vi "Lab Panel V4.83.vi"() -> ()   [LabVIEW 2013] (continued)
            n215 = property on="Network Directory" class="Path"("Blinking"=w253) -> ()  [unwired: 2 in, 2 out]
            n216 = property on="Message" class="Str"("Blinking"=w253) -> ()  [unwired: 2 in, 2 out]
          }
        }
        frame #10 {
          w261 = FALSE
          n217 = property on="Message" class="Str"("Blinking"=w261) -> ()  [unwired: 2 in, 2 out]
          n218 = property on="Network Directory" class="Path"("Blinking"=w261) -> ()  [unwired: 2 in, 2 out]
          n219 = property on="Tab Control 2" class="TabCtl (strict)"("Value"=0) -> ()  [unwired: 2 in, 2 out]
        }
      }
    }
    frame #2 {
      n220 = node-c288("loop  delay(mS)") -> (w265:T15)  [unwired: 3 in]
      n221 = timed-loop {
        timing: w265 -> [_]
        timing-out: [_] -> w264
        i -> [w287]
        stop <- "stop" stop-if-true
        n222 = node-c288() -> ()  [unwired: 1 in, 1 out]
        n223 = global write "Global display 1.vi" "stop disp"("stop") -> ()
        n224 = local read "SELECT LAB05-2"() -> (w267:T3)
        n225 = local read "SELECT LAB05-1"() -> (w268:T3)
        n226 = local read "SELECT LAB04-2"() -> (w269:T3)
        n227 = local read "SELECT LAB03-1"() -> (w272:T3)
        n228 = local read "SELECT LAB02-2"() -> (w273:T3)
        n229 = local read "SELECT LAB01-1"() -> (w276:T3)
        n230 = local read "SELECT LAB03-2"() -> (w271:T3)
        n231 = local read "SELECT LAB01-2"() -> (w275:T3)
        n232 = local read "SELECT LAB04-1"() -> (w270:T3)
        n233 = local read "SELECT LAB02-1"() -> (w274:T3)
        n234 = local read "run lab03-2"() -> (w281:bool)
        n235 = local read "run lab04-1"() -> (w280:bool)
        n236 = local read "run lab05-1"() -> (w278:bool)
        n237 = local read "run lab04-2"() -> (w279:bool)
        n238 = local read "run lab05-2"() -> (w277:bool)
        n239 = local read "run lab03-1"() -> (w282:bool)
        n240 = local read "run lab02-2"() -> (w283:bool)
        n241 = local read "run lab02-1"() -> (w284:bool)
        n242 = local read "run lab01-1"() -> (w286:bool)
        n243 = local read "run lab01-2"() -> (w285:bool)
        n244 = stacked-sequence {
          seq-local: [_ w349 _ _ _ _ _ _ _ _ _ _ _ _ _ _ _ _ _ _ _] -> [_ _ _ _ _ w1958 _ _ _ _ _ _ _ _ _ _ _ _ _ _ _]
          seq-local: [_ w348 _ _ _ _ _ _ _ _ _ _ _ _ _ _ _ _ _ _ _] -> [_ _ _ _ _ w1957 _ _ _ _ _ _ _ _ _ _ _ _ _ _ _]
          seq-local: [_ w335 _ _ _ _ _ _ _ _ _ _ _ _ _ _ _ _ _ _ _] -> [_ _ _ _ _ w1956 _ _ _ _ _ _ _ _ _ _ _ _ _ _ _]
          seq-local: [_ w334 _ _ _ _ _ _ _ _ _ _ _ _ _ _ _ _ _ _ _] -> [_ _ _ _ _ w1955 _ _ _ _ _ _ _ _ _ _ _ _ _ _ _]
          seq-local: [_ w333 _ _ _ _ _ _ _ _ _ _ _ _ _ _ _ _ _ _ _] -> [_ _ _ _ _ w1954 _ _ _ _ _ _ _ _ _ _ _ _ _ _ _]
          seq-local: [_ w332 _ _ _ _ _ _ _ _ _ _ _ _ _ _ _ _ _ _ _] -> [_ _ _ _ _ w1953 _ _ _ _ _ _ _ _ _ _ _ _ _ _ _]
          seq-local: [_ w331 _ _ _ _ _ _ _ _ _ _ _ _ _ _ _ _ _ _ _] -> [_ _ _ _ _ w1952 _ _ _ _ _ _ _ _ _ _ _ _ _ _ _]
          seq-local: [_ w330 _ _ _ _ _ _ _ _ _ _ _ _ _ _ _ _ _ _ _] -> [_ _ _ _ _ w1951 _ _ _ _ _ _ _ _ _ _ _ _ _ _ _]
          seq-local: [_ w329 _ _ _ _ _ _ _ _ _ _ _ _ _ _ _ _ _ _ _] -> [_ _ _ _ _ w1950 _ _ _ _ _ _ _ _ _ _ _ _ _ _ _]
          seq-local: [_ w328 _ _ _ _ _ _ _ _ _ _ _ _ _ _ _ _ _ _ _] -> [_ _ _ _ _ w1949 _ _ _ _ _ _ _ _ _ _ _ _ _ _ _]
          tunnel: w286 -> [_ _ w365 w604 w1548 w1978 w2288 w2533 _ _ _ _ w2936 _ w3864 _ _ w4147 w4450 w4623 _]
          tunnel: w285 -> [_ _ w364 w602 w1547 w1977 w2289 w2532 _ _ _ _ w2935 _ w3862 _ _ w4146 w4449 w4621 _]
          tunnel: w284 -> [_ _ w363 w600 w1546 w1976 w2287 w2531 _ _ _ _ w2934 _ w3860 _ _ w4145 w4448 _ _]
          tunnel: w283 -> [_ _ w362 w598 w1545 w1975 w2286 w2530 _ _ _ _ w2933 _ w3858 _ _ w4144 w4447 _ _]
          tunnel: w282 -> [_ _ w361 w596 w1544 w1974 w2285 w2529 _ _ _ _ w2932 _ w3856 _ _ w4143 w4446 _ _]
          tunnel: w281 -> [_ _ w360 w594 w1543 w1973 w2284 w2528 _ _ _ _ w2931 _ w3854 _ _ w4142 w4445 _ _]
          tunnel: w280 -> [_ _ w359 w592 w1542 w1972 w2283 w2527 _ _ _ _ w2930 _ w3852 _ _ w4141 w4444 _ _]
          tunnel: w279 -> [_ _ w358 w590 w1541 w1971 w2282 w2526 _ _ _ _ w2929 _ w3850 _ _ w4140 w4443 _ _]
          tunnel: w278 -> [_ _ w357 w588 w1540 w1970 w2281 w2525 _ _ _ _ w2928 _ w3848 _ _ w4139 w4442 _ _]
          tunnel: w277 -> [_ _ w356 w586 w1539 w1969 w2280 w2524 _ _ _ _ w2927 _ w3846 _ _ w4138 w4441 _ _]
          tunnel: w276 -> [_ _ _ w603 w1538 w1968 _ _ _ _ _ _ _ _ w3866 _ _ _ _ _ _]
          tunnel: w275 -> [_ _ _ w601 w1537 w1967 _ _ _ _ _ _ _ _ w3861 _ _ _ _ _ _]
          tunnel: w274 -> [_ _ _ w599 w1536 w1966 _ _ _ _ _ _ _ _ w3859 _ _ _ _ _ _]
          tunnel: w273 -> [_ _ _ w597 w1535 w1965 _ _ _ _ _ _ _ _ w3857 _ _ _ _ _ _]
          tunnel: w272 -> [_ _ _ w595 w1534 w1964 _ _ _ _ _ _ _ _ w3855 _ _ _ _ _ _]
          tunnel: w271 -> [_ _ _ w593 w1533 w1963 _ _ _ _ _ _ _ _ w3853 _ _ _ _ _ _]
          tunnel: w270 -> [_ _ _ w591 w1532 w1962 _ _ _ _ _ _ _ _ w3851 _ _ _ _ _ _]
          tunnel: w269 -> [_ _ _ w589 w1531 w1961 _ _ _ _ _ _ _ _ w3849 _ _ _ _ _ _]
          tunnel: w268 -> [_ _ _ w587 w1530 w1960 _ _ _ _ _ _ _ _ w3847 _ _ _ _ _ _]
          tunnel: w267 -> [_ _ _ w585 w1529 w1959 _ _ _ _ _ _ _ _ w3845 _ _ _ _ _ _]
          frame #0 {
            w291 = FALSE
            w296 = 0.5
            # "set up cycle control"
            n245 = local read "jig cycle"() -> (w295:dbl)
            n246 = Divide(x="JIG ON TIME (S)", y=w296) -> (x/y=→"on loops":dbl)
            n247 = Divide(x="JIG OFF TIME (S)", y=w296) -> (x/y=→"off loops":dbl)
            n248 = Increment(x=w295) -> (x+1=w294:dbl)
            n249 = local write "TEMP"(w291) -> ()
            n250 = local write "AI"(w291) -> ()
            n251 = local write "jig cycle"(w294) -> ()
            n252 = event shown="[1] \"ADMIN\": Value Change" {
              selector: _ -> [_ _]
              dyn-events: _ -> [_ _]
              timeout: 10 -> [_ _]
              event Timeout {
                n253 = event-data() -> ()  [unwired: 1 in, 3 out]
              }
              event "ADMIN": Value Change {
                n254 = event-data() -> ()  [unwired: 1 in, 6 out]
                n255 = stacked-sequence {
                  seq-local: [_ w300 _] -> [_ _ w301]
                  frame #0 {
                    n256 = global write "Global 1.vi" "password"("9999") -> ()
                  }
                  frame #1 {
                    n257 = call "sub vi - password 1.vi"() -> ("RESULT"=w300:bool)  [unwired: 11 in]
                  }
                  frame #2 {
                    w303 = FALSE
                    n258 = property on="Tab Control 2" class="TabCtl (strict)"() -> ("Pages"=w307:refnum<vi>[])  [unwired: 2 in, 2 out]
                    n259 = Select(t=TRUE, s=w301, f=w303) -> (s? t:f=w302:bool)
                    n260 = Index Array(array=w307, index=9) -> (element=w305:refnum<vi>)
                    n261 = property class="Page"(reference=w305, "PageVis"=w302) -> ()  [unwired: 1 in, 2 out]
                    n262 = local write "ADMIN"(w303) -> ()
                  }
                }
              }
            }
          }
          frame #1 {
            w345 = 60.0
            # "convert temperature rise minutes to cycles"
            n263 = local read "SET LAB05-2"() -> (w309:T5)
            n264 = local read "SET LAB05-1"() -> (w311:T5)
            n265 = local read "SET LAB04-2"() -> (w313:T5)
            n266 = local read "SET LAB01-1"() -> (w327:T5)
            n267 = local read "SET LAB01-2"() -> (w325:T5)
            n268 = local read "SET LAB02-2"() -> (w321:T5)
            n269 = local read "SET LAB04-1"() -> (w315:T5)
            n270 = local read "SET LAB03-1"() -> (w319:T5)
            n271 = local read "SET LAB03-2"() -> (w317:T5)
            n272 = local read "SET LAB02-1"() -> (w323:T5)
            n273 = local read "JIG OFF TIME (S)"() -> (w350:dbl)
            n274 = local read "JIG ON TIME (S)"() -> (w351:dbl)
            n275 = Unbundle(w309) -> ("T-RISE mins"=w308:dbl)  [unwired: 4 out]
            n276 = Unbundle(w311) -> ("T-RISE mins"=w310:dbl)  [unwired: 4 out]
            n277 = Unbundle(w327) -> ("T-RISE mins"=w326:dbl)  [unwired: 4 out]
            n278 = Unbundle(w313) -> ("T-RISE mins"=w312:dbl)  [unwired: 4 out]
            n279 = Unbundle(w325) -> ("T-RISE mins"=w324:dbl)  [unwired: 4 out]
            n280 = Unbundle(w323) -> ("T-RISE mins"=w322:dbl)  [unwired: 4 out]
            n281 = Unbundle(w315) -> ("T-RISE mins"=w314:dbl)  [unwired: 4 out]
            n282 = Unbundle(w321) -> ("T-RISE mins"=w320:dbl)  [unwired: 4 out]
            n283 = Unbundle(w317) -> ("T-RISE mins"=w316:dbl)  [unwired: 4 out]
            n284 = Unbundle(w319) -> ("T-RISE mins"=w318:dbl)  [unwired: 4 out]
            n285 = Add(x=w351, y=w350) -> (x+y=w344:dbl)
            n286 = Multiply(x=w345, y=w316) -> (x*y=w340:dbl)
            n287 = Multiply(x=w345, y=w314) -> (x*y=w339:dbl)
            n288 = Multiply(x=w345, y=w312) -> (x*y=w338:dbl)
            n289 = Multiply(x=w345, y=w310) -> (x*y=w337:dbl)
            n290 = Multiply(x=w345, y=w308) -> (x*y=w336:dbl)
            n291 = Multiply(x=w345, y=w324) -> (x*y=w346:dbl)
            n292 = Multiply(x=w345, y=w318) -> (x*y=w341:dbl)
            n293 = Multiply(x=w345, y=w326) -> (x*y=w347:dbl)
            n294 = Multiply(x=w345, y=w322) -> (x*y=w343:dbl)
            n295 = Multiply(x=w345, y=w320) -> (x*y=w342:dbl)
            n296 = Divide(x=w337, y=w344) -> (x/y=w329:dbl)
            n297 = Divide(x=w338, y=w344) -> (x/y=w330:dbl)
            n298 = Divide(x=w339, y=w344) -> (x/y=w331:dbl)
            n299 = Divide(x=w336, y=w344) -> (x/y=w328:dbl)
            n300 = Divide(x=w341, y=w344) -> (x/y=w333:dbl)
            n301 = Divide(x=w347, y=w344) -> (x/y=w349:dbl)
            n302 = Divide(x=w346, y=w344) -> (x/y=w348:dbl)
            n303 = Divide(x=w343, y=w344) -> (x/y=w335:dbl)
            n304 = Divide(x=w342, y=w344) -> (x/y=w334:dbl)
            n305 = Divide(x=w340, y=w344) -> (x/y=w332:dbl)
          }
          frame #2 {
            # "control cycle loops"
            n306 = local read "JIG OFF TIME (S)"() -> (w354:dbl)
            n307 = local read "JIG ON TIME (S)"() -> (w353:dbl)
            n308 = local read "jig cycle"() -> (w367:dbl)
            n309 = local read "on loops"() -> (w369:dbl)
            n310 = local read "off loops"() -> (w368:dbl)
            n311 = Add(x=w354, y=w353) -> (x+y=w352:dbl)
            n312 = Add(x=w369, y=w368) -> (x+y=w355:dbl)
            n313 = Greater Or Equal?(x=w367, y=w355) -> (x >= y?=w366:bool)
            n314 = case shown="True" w366 {
              tunnel: w365 -> [_ w404]
              tunnel: w364 -> [_ w403]
              tunnel: w363 -> [_ w402]
              tunnel: w362 -> [_ w401]
              tunnel: w361 -> [_ w400]
              tunnel: w360 -> [_ w399]
              tunnel: w359 -> [_ w398]
              tunnel: w358 -> [_ w397]
              tunnel: w357 -> [_ w396]
              tunnel: w356 -> [_ w395]
              tunnel: w352 -> [_ w394]
              frame False {
              }
              frame True {
                # "increment cycle value and convert cycles to minutes for temp rise"
                n315 = local read "Temp Loops"() -> (w371:dbl)
                n316 = local read "JIG RELAY CYCLES"() -> (w393:T7)
                n317 = Increment(x=w371) -> (x+1=w370:dbl)
                n318 = local write "Temp Loops"(w370) -> ()
                n319 = Unbundle By Name(w393) -> ("LAB01-1"=w391:dbl, "LAB01-2"=w389:dbl, "LAB02-1"=w387:dbl, "LAB02-2"=w385:dbl, "LAB03-1"=w383:dbl, "LAB03-2"=w381:dbl, "LAB04-1"=w379:dbl, "LAB04-2"=w377:dbl, "LAB05-1"=w375:dbl, "LAB05-2"=w373:dbl)
                n320 = stacked-sequence {
                  tunnel: w404 -> [w416 _ _ _ _ _ _ _ _ _]
                  tunnel: w403 -> [_ w433 _ _ _ _ _ _ _ _]
                  tunnel: w402 -> [_ _ w450 _ _ _ _ _ _ _]
                  tunnel: w401 -> [_ _ _ w467 _ _ _ _ _ _]
                  tunnel: w400 -> [_ _ _ _ w484 _ _ _ _ _]
                  tunnel: w399 -> [_ _ _ _ _ w501 _ _ _ _]
                  tunnel: w398 -> [_ _ _ _ _ _ w518 _ _ _]
                  tunnel: w397 -> [_ _ _ _ _ _ _ w535 _ _]
                  tunnel: w396 -> [_ _ _ _ _ _ _ _ w552 _]
                  tunnel: w395 -> [_ _ _ _ _ _ _ _ _ w569]
                  tunnel: w394 -> [w413 w430 w447 w464 w481 w498 w515 w532 w549 w566]
                  tunnel: w391 -> [w407 _ _ _ _ _ _ _ _ _]
                  tunnel: [w406 _ _ _ _ _ _ _ _ _] -> w390
                  tunnel: w389 -> [_ w424 _ _ _ _ _ _ _ _]
                  tunnel: [_ w423 _ _ _ _ _ _ _ _] -> w388
                  tunnel: w387 -> [_ _ w441 _ _ _ _ _ _ _]
                  tunnel: [_ _ w440 _ _ _ _ _ _ _] -> w386
                  tunnel: w385 -> [_ _ _ w458 _ _ _ _ _ _]
                  tunnel: [_ _ _ w457 _ _ _ _ _ _] -> w384
                  tunnel: w383 -> [_ _ _ _ w475 _ _ _ _ _]
                  tunnel: [_ _ _ _ w474 _ _ _ _ _] -> w382
                  tunnel: w381 -> [_ _ _ _ _ w492 _ _ _ _]
                  tunnel: [_ _ _ _ _ w491 _ _ _ _] -> w380
                  tunnel: w379 -> [_ _ _ _ _ _ w509 _ _ _]
                  tunnel: [_ _ _ _ _ _ w508 _ _ _] -> w378
                  tunnel: w377 -> [_ _ _ _ _ _ _ w526 _ _]
                  tunnel: [_ _ _ _ _ _ _ w525 _ _] -> w376
                  tunnel: w375 -> [_ _ _ _ _ _ _ _ w543 _]
                  tunnel: [_ _ _ _ _ _ _ _ w542 _] -> w374
                  tunnel: w373 -> [_ _ _ _ _ _ _ _ _ w560]
                  tunnel: [_ _ _ _ _ _ _ _ _ w559] -> w372
                  frame #0 {
                    n321 = local read "DISP LAB01-1"() -> (w411:T4)
                    n322 = Unbundle(w411) -> ("CYCLE"=w412:dbl)  [unwired: 2 out]
                    n323 = case shown="True" w416 {
                      tunnel: w412 -> [w418 w422]
                      tunnel: [w418 w421] -> w410
                      tunnel: w407 -> [w417 w420]
                      tunnel: [w417 w419] -> w406
                      frame False {
                      }
                      frame True {
                        n324 = Increment(x=w420) -> (x+1=w419:dbl)
                        n325 = Increment(x=w422) -> (x+1=w421:dbl)
                      }
                    }
                    n326 = Multiply(x=w410, y=w413) -> (x*y=w414:dbl)
                    n327 = Divide(x=w414, y=60.0) -> (x/y=w409:dbl)
                    n328 = Bundle(cluster=w411, "CYCLE"=w410, "MINS"=w409) -> (w408:T4)  [unwired: 1 in]
                    n329 = local write "DISP LAB01-1"(w408) -> ()
                  }
                  frame #1 {
                    n330 = local read "DISP LAB01-2"() -> (w428:T4)
                    n331 = Unbundle(w428) -> ("CYCLE"=w429:dbl)  [unwired: 2 out]
                    n332 = case shown="True" w433 {
                      tunnel: w429 -> [w435 w439]
                      tunnel: [w435 w438] -> w426
                      tunnel: w424 -> [w434 w437]
                      tunnel: [w434 w436] -> w423
                      frame False {
                      }
                      frame True {
                        n333 = Increment(x=w437) -> (x+1=w436:dbl)
                        n334 = Increment(x=w439) -> (x+1=w438:dbl)
                      }
                    }
                    n335 = Multiply(x=w426, y=w430) -> (x*y=w431:dbl)
                    n336 = Divide(x=w431, y=60.0) -> (x/y=w425:dbl)
                    n337 = Bundle(cluster=w428, "CYCLE"=w426, "MINS"=w425) -> (w427:T4)  [unwired: 1 in]
                    n338 = local write "DISP LAB01-2"(w427) -> ()
                  }
                  frame #2 {
                    n339 = local read "DISP LAB02-1"() -> (w445:T4)
                    n340 = Unbundle(w445) -> ("CYCLE"=w446:dbl)  [unwired: 2 out]
                    n341 = case shown="True" w450 {
                      tunnel: [w452 w456] -> w443
                      tunnel: w446 -> [w452 w455]
                      tunnel: w441 -> [w451 w454]
                      tunnel: [w451 w453] -> w440
                      frame False {
                      }
                      frame True {
                        n342 = Increment(x=w454) -> (x+1=w453:dbl)
                        n343 = Increment(x=w455) -> (x+1=w456:dbl)
                      }
                    }
                    n344 = Multiply(x=w443, y=w447) -> (x*y=w448:dbl)
                    n345 = Divide(x=w448, y=60.0) -> (x/y=w442:dbl)
                    n346 = Bundle(cluster=w445, "CYCLE"=w443, "MINS"=w442) -> (w444:T4)  [unwired: 1 in]
                    n347 = local write "DISP LAB02-1"(w444) -> ()
                  }
                  frame #3 {
                    n348 = local read "DISP LAB02-2"() -> (w462:T4)
                    n349 = Unbundle(w462) -> ("CYCLE"=w463:dbl)  [unwired: 2 out]
                    n350 = case shown="True" w467 {
                      tunnel: [w469 w473] -> w461
                      tunnel: w463 -> [w469 w472]
                      tunnel: w458 -> [w468 w471]
                      tunnel: [w468 w470] -> w457
                      frame False {
                      }
                      frame True {
                        n351 = Increment(x=w471) -> (x+1=w470:dbl)
                        n352 = Increment(x=w472) -> (x+1=w473:dbl)
                      }
                    }
                    n353 = Multiply(x=w461, y=w464) -> (x*y=w465:dbl)
                    n354 = Divide(x=w465, y=60.0) -> (x/y=w460:dbl)
                    n355 = Bundle(cluster=w462, "CYCLE"=w461, "MINS"=w460) -> (w459:T4)  [unwired: 1 in]
                    n356 = local write "DISP LAB02-2"(w459) -> ()
                  }
                  frame #4 {
                    n357 = local read "DISP LAB03-1"() -> (w479:T4)
                    n358 = Unbundle(w479) -> ("CYCLE"=w480:dbl)  [unwired: 2 out]
                    n359 = case shown="True" w484 {
                      tunnel: [w486 w490] -> w476
                      tunnel: w480 -> [w486 w489]
                      tunnel: w475 -> [w485 w488]
                      tunnel: [w485 w487] -> w474
                      frame False {
                      }
                      frame True {
                        n360 = Increment(x=w488) -> (x+1=w487:dbl)
                        n361 = Increment(x=w489) -> (x+1=w490:dbl)
                      }
                    }
                    n362 = Multiply(x=w476, y=w481) -> (x*y=w482:dbl)
                    n363 = Divide(x=w482, y=60.0) -> (x/y=w477:dbl)
                    n364 = Bundle(cluster=w479, "CYCLE"=w476, "MINS"=w477) -> (w478:T4)  [unwired: 1 in]
                    n365 = local write "DISP LAB03-1"(w478) -> ()
                  }
                  frame #5 {
                    n366 = local read "DISP LAB03-2"() -> (w496:T4)
                    n367 = Unbundle(w496) -> ("CYCLE"=w497:dbl)  [unwired: 2 out]
                    n368 = case shown="True" w501 {
                      tunnel: [w503 w507] -> w495
                      tunnel: w497 -> [w503 w506]
                      tunnel: w492 -> [w502 w505]
                      tunnel: [w502 w504] -> w491
                      frame False {
                      }
                      frame True {
                        n369 = Increment(x=w505) -> (x+1=w504:dbl)
                        n370 = Increment(x=w506) -> (x+1=w507:dbl)
                      }
                    }
                    n371 = Multiply(x=w495, y=w498) -> (x*y=w499:dbl)
                    n372 = Divide(x=w499, y=60.0) -> (x/y=w494:dbl)
                    n373 = Bundle(cluster=w496, "CYCLE"=w495, "MINS"=w494) -> (w493:T4)  [unwired: 1 in]
                    n374 = local write "DISP LAB03-2"(w493) -> ()
                  }
                  frame #6 {
                    n375 = local read "DISP LAB04-1"() -> (w513:T4)
                    n376 = Unbundle(w513) -> ("CYCLE"=w514:dbl)  [unwired: 2 out]
                    n377 = case shown="True" w518 {
                      tunnel: [w520 w524] -> w511
                      tunnel: w514 -> [w520 w523]
                      tunnel: w509 -> [w519 w522]
                      tunnel: [w519 w521] -> w508
                      frame False {
                      }
                      frame True {
                        n378 = Increment(x=w522) -> (x+1=w521:dbl)
                        n379 = Increment(x=w523) -> (x+1=w524:dbl)
                      }
                    }
                    n380 = Multiply(x=w511, y=w515) -> (x*y=w516:dbl)
                    n381 = Divide(x=w516, y=60.0) -> (x/y=w510:dbl)
                    n382 = Bundle(cluster=w513, "CYCLE"=w511, "MINS"=w510) -> (w512:T4)  [unwired: 1 in]
                    n383 = local write "DISP LAB04-1"(w512) -> ()
                  }
                  frame #7 {
                    n384 = local read "DISP LAB04-2"() -> (w530:T4)
                    n385 = Unbundle(w530) -> ("CYCLE"=w531:dbl)  [unwired: 2 out]
                    n386 = case shown="True" w535 {
                      tunnel: [w537 w541] -> w528
                      tunnel: w531 -> [w537 w540]
                      tunnel: w526 -> [w536 w539]
                      tunnel: [w536 w538] -> w525
                      frame False {
                      }
                      frame True {
                        n387 = Increment(x=w539) -> (x+1=w538:dbl)
                        n388 = Increment(x=w540) -> (x+1=w541:dbl)
                      }
                    }
                    n389 = Multiply(x=w528, y=w532) -> (x*y=w534:dbl)
                    n390 = Divide(x=w534, y=60.0) -> (x/y=w527:dbl)
                    n391 = Bundle(cluster=w530, "CYCLE"=w528, "MINS"=w527) -> (w529:T4)  [unwired: 1 in]
                    n392 = local write "DISP LAB04-2"(w529) -> ()
                  }
                  frame #8 {
                    n393 = local read "DISP LAB05-1"() -> (w547:T4)
                    n394 = Unbundle(w547) -> ("CYCLE"=w548:dbl)  [unwired: 2 out]
                    n395 = case shown="True" w552 {
                      tunnel: [w554 w558] -> w545
                      tunnel: w548 -> [w554 w557]
                      tunnel: w543 -> [w553 w556]
                      tunnel: [w553 w555] -> w542
                      frame False {
                      }
                      frame True {
                        n396 = Increment(x=w556) -> (x+1=w555:dbl)
                        n397 = Increment(x=w557) -> (x+1=w558:dbl)
                      }
                    }
                    n398 = Multiply(x=w545, y=w549) -> (x*y=w550:dbl)
                    n399 = Divide(x=w550, y=60.0) -> (x/y=w544:dbl)
                    n400 = Bundle(cluster=w547, "CYCLE"=w545, "MINS"=w544) -> (w546:T4)  [unwired: 1 in]
                    n401 = local write "DISP LAB05-1"(w546) -> ()
                  }
                  frame #9 {
                    n402 = local read "DISP LAB05-2"() -> (w565:T4)
                    n403 = Unbundle(w565) -> ("CYCLE"=w564:dbl)  [unwired: 2 out]
                    n404 = case shown="True" w569 {
                      tunnel: [w571 w575] -> w563
                      tunnel: w564 -> [w571 w574]
                      tunnel: w560 -> [w570 w573]
                      tunnel: [w570 w572] -> w559
                      frame False {
                      }
                      frame True {
                        n405 = Increment(x=w573) -> (x+1=w572:dbl)
                        n406 = Increment(x=w574) -> (x+1=w575:dbl)
                      }
                    }
                    n407 = Multiply(x=w563, y=w566) -> (x*y=w567:dbl)
                    n408 = Divide(x=w567, y=60.0) -> (x/y=w562:dbl)
                    n409 = Bundle(cluster=w565, "CYCLE"=w563, "MINS"=w562) -> (w561:T4)  [unwired: 1 in]
                    n410 = local write "DISP LAB05-2"(w561) -> ()
                  }
                }
                n411 = local write "jig cycle"(0) -> ()
                n412 = Bundle By Name(cluster=w393, "LAB01-1"=w390, "LAB01-2"=w388, "LAB02-1"=w386, "LAB02-2"=w384, "LAB03-1"=w382, "LAB03-2"=w380, "LAB04-1"=w378, "LAB04-2"=w376, "LAB05-1"=w374, "LAB05-2"=w372) -> (w392:T7)
                n413 = local write "JIG RELAY CYCLES"(w392) -> ()
              }
            }
          }
          frame #3 {
            # "START & STOP test RUN switch change, start test if true and stop test if false"
            n414 = Get Date/Time In Seconds() -> (seconds since 1Jan1904=w583:timestamp)
            n415 = local read "C drive data root dir"() -> (w576:path)
            n416 = Format Date/Time String(time format string (%c)="%b\\%a%d", seconds (now)=w583) -> (date/time string=w607:string)  [unwired: 1 in]
            n417 = Format Date/Time String(time format string (%c)="%H%M", seconds (now)=w583) -> (date/time string=w605:string)  [unwired: 1 in]
            n418 = Format Date/Time String(time format string (%c)="LabPanel%Y", seconds (now)=w583) -> (date/time string=w582:string)  [unwired: 1 in]
            n419 = Path To String(path=w576) -> (string=w579:string)
            n420 = global write "Global 1.vi" "C drive root path"(w576) -> ()
            n421 = Concatenate Strings(w579, "\\") -> (w577:string)
            n422 = event shown="[5] \"RUN LAB03-1\": Value Change" {
              selector: _ -> [_ _ _ _ _ _ _ _ _ _ _]
              dyn-events: _ -> [_ _ _ _ _ _ _ _ _ _ _]
              timeout: 10 -> [_ _ _ _ _ _ _ _ _ _ _]
              tunnel: w577 -> [_ w615 w707 w799 w891 w983 w1075 w1167 w1259 w1351 w1443]
              tunnel: w607 -> [_ w614 w706 w798 w890 w982 w1074 w1166 w1258 w1350 w1442]
              tunnel: w605 -> [_ w612 w705 w797 w889 w981 w1073 w1165 w1257 w1349 w1441]
              tunnel: w603 -> [_ w613 _ _ _ _ _ _ _ _ _]
              tunnel: w604 -> [_ _ _ _ _ _ _ _ _ _ _]
              tunnel: w602 -> [_ _ _ _ _ _ _ _ _ _ _]
              tunnel: w601 -> [_ _ w704 _ _ _ _ _ _ _ _]
              tunnel: w600 -> [_ _ _ _ _ _ _ _ _ _ _]
              tunnel: w599 -> [_ _ _ w796 _ _ _ _ _ _ _]
              tunnel: w598 -> [_ _ _ _ _ _ _ _ _ _ _]
              tunnel: w597 -> [_ _ _ _ w888 _ _ _ _ _ _]
              tunnel: w596 -> [_ _ _ _ _ _ _ _ _ _ _]
              tunnel: w595 -> [_ _ _ _ _ w980 _ _ _ _ _]
              tunnel: w594 -> [_ _ _ _ _ _ _ _ _ _ _]
              tunnel: w593 -> [_ _ _ _ _ _ w1072 _ _ _ _]
              tunnel: w592 -> [_ _ _ _ _ _ _ _ _ _ _]
              tunnel: w591 -> [_ _ _ _ _ _ _ w1164 _ _ _]
              tunnel: w590 -> [_ _ _ _ _ _ _ _ _ _ _]
              tunnel: w589 -> [_ _ _ _ _ _ _ _ w1256 _ _]
              tunnel: w588 -> [_ _ _ _ _ _ _ _ _ _ _]
              tunnel: w587 -> [_ _ _ _ _ _ _ _ _ w1348 _]
              tunnel: w586 -> [_ _ _ _ _ _ _ _ _ _ _]
              tunnel: w585 -> [_ _ _ _ _ _ _ _ _ _ w1440]
              tunnel: w582 -> [_ w611 w703 w795 w887 w979 w1071 w1163 w1255 w1347 w1439]
              tunnel: [_ w610 w702 w794 w886 w978 w1070 w1162 w1254 w1346 w1438] -> w580
              event Timeout {
                n423 = event-data() -> ()  [unwired: 1 in, 3 out]
              }
              event "RUN LAB01-1": Value Change {
                n424 = event-data() -> ("NewVal"=w609:bool)  [unwired: 1 in, 5 out]
                n425 = local write "run lab01-1"(w609) -> ()
                n426 = case shown="True" w609 {
                  tunnel: w615 -> [_ w648]
                  tunnel: w614 -> [_ w647]
                  tunnel: w613 -> [w617 w646]
                  tunnel: w612 -> [_ w645]
                  tunnel: w611 -> [_ w644]
                  tunnel: [w616 w643] -> w610
                  frame False {
                    # "stop test"
                    n427 = stacked-sequence {
                      tunnel: w617 -> [_ w629 _ _]
                      tunnel: [_ w621 _ _] -> w616
                      frame #0 {
                        n428 = local read "DISP LAB01-1"() -> (w620:T4)
                        n429 = Bundle(cluster=w620, "STATUS"="STOP") -> (w618:T4)  [unwired: 2 in]
                        n430 = local write "DISP LAB01-1"(w618) -> ()
                      }
                      frame #1 {
                        n431 = local read "DISP LAB01-1"() -> (w628:T4)
                        n432 = Unbundle(w628) -> ("CYCLE"=w626:dbl, "MINS"=w627:dbl)  [unwired: 1 out]
                        n433 = case shown="\"CYCLE TEST\"" w629 {
                          tunnel: w627 -> [_ _ w636]
                          tunnel: w626 -> [w634 w635 _]
                          tunnel: [w634 w635 w636] -> w625
                          frame "CHART TEST", Default {
                          }
                          frame "CYCLE TEST" {
                          }
                          frame "T-RISE TEST" {
                          }
                        }
                        n434 = local read "TDMS LAB01-1"() -> (w633:refnum<k34>)
                        n435 = Build Array("STOPPED") -> (w630:string[])
                        n436 = Build Array(w625) -> (w624:dbl[])
                        n437 = TDMS Write(0:w633, 5:"TEST RESULT", 7:w630, 9:w624) -> (4:w622:refnum<k34>, 15:w623:errorcluster)  [unwired: 2 in, 2 out]
                        n438 = TDMS Close(8:w623, 11:w622) -> (0:w621:errorcluster)  [unwired: 1 out]
                      }
                      frame #2 {
                        n439 = stacked-sequence {
                          tunnel: "LAB01-1" -> [w639 w641]
                          frame #0 {
                            n440 = call "sub vi - defrag tdms v1.vi"("panel id"=w639) -> ("error out"=w638:errorcluster)  [unwired: 10 in]
                            n441 = local write "data file error"(w638) -> ()
                          }
                          frame #1 {
                            n442 = call "Save data file to network drive v1.vi"("panel id"=w641) -> ("network file save error"=w640:errorcluster)  [unwired: 9 in, 1 out]
                            n443 = local write "RESULT LAB01-1"(FALSE) -> ()
                            n444 = local write "data file error"(w640) -> ()
                          }
                        }
                      }
                      frame #3 {
                      }
                    }
                  }
                  frame True {
                    # "start new test and create test file"
                    n445 = stacked-sequence {
                      seq-local: [w649 _ _ _ _] -> [_ w670 _ _ _]
                      tunnel: w648 -> [w654 _ _ _ _]
                      tunnel: w647 -> [w650 _ _ _ _]
                      tunnel: w646 -> [w664 _ _ _ _]
                      tunnel: w645 -> [w657 _ _ _ _]
                      tunnel: w644 -> [w652 _ _ _ _]
                      tunnel: [_ w671 _ _ _] -> w643
                      frame #0 {
                        w651 = "\\"
                        n446 = case shown="\"CHART TEST\", Default" w664 {
                          tunnel: ["L01-1-CHART TEST-" "L01-1-CYCLE TEST-" "L01-1-T-RISE TEST-"] -> w660
                          frame "CHART TEST", Default {
                          }
                          frame "CYCLE TEST" {
                          }
                          frame "T-RISE TEST" {
                          }
                        }
                        n447 = local read "SET LAB01-1"() -> (w659:T5)
                        n448 = Unbundle(w659) -> ("DESCRIPTION"=w658:string)  [unwired: 4 out]
                        n449 = Concatenate Strings(w654, "\\", w652, w651, w650, w651) -> (w661:string)
                        n450 = String To Path(string=w661) -> (path=w663:path)
                        n451 = Concatenate Strings(w661, w660, w658, "-", w657, ".tdms") -> (w649:string)
                        n452 = Create Folder(path (use dialog)=w663) -> (error out=w662:errorcluster)  [unwired: 2 in, 2 out]
                        n453 = call <vilib>:"Clear Errors.vi"("error in (no error)"=w662) -> ()  [unwired: 6 in, 1 out]
                        n454 = global write "Global 1.vi" "LAB01-1 FILE"(w649) -> ()
                      }
                      frame #1 {
                        n455 = String To Path(string=w670) -> (path=w668:path)
                        n456 = TDMS Open(5:FALSE, 6:FALSE, 10:T18."create or replace" ("operation (0:open)"), 11:w668) -> (0:w671:errorcluster, 3:→"TDMS LAB01-1":refnum<k34>)  [unwired: 3 in]
                      }
                      frame #2 {
                        n457 = local read "TDMS LAB01-1"() -> (w691:refnum<k34>)
                        n458 = local read "SET LAB01-1"() -> (w680:T5)
                        n459 = Build Array("Testers Name", "Description", "Set Test Cycles", "T-Rise minutes", "T-Rise Deg C") -> (w681:string[])
                        n460 = Unbundle(w680) -> ("NAME"=w679:string, "DESCRIPTION"=w678:string, "CYCLES"=w677:dbl, "T-RISE mins"=w676:dbl, "T-RISE deg C"=w675:dbl)
                        n461 = Number To Decimal String(number=w677) -> (decimal integer string=w690:string)  [unwired: 1 in]
                        n462 = Number To Decimal String(number=w676) -> (decimal integer string=w689:string)  [unwired: 1 in]
                        n463 = Number To Decimal String(number=w675) -> (decimal integer string=w688:string)  [unwired: 1 in]
                        n464 = Build Array(w679, w678, w690, w689, w688) -> (w687:string[])
                        n465 = TDMS Set Properties(5:w687, 7:w681, 11:w691) -> ()  [unwired: 3 in, 4 out]
                      }
                      frame #3 {
                        w692 = 0.0
                        n466 = local read "DISP LAB01-1"() -> (w695:T4)
                        n467 = Bundle(cluster=w695, "CYCLE"=w692, "MINS"=w692, "STATUS"="RUN") -> (w694:T4)
                        n468 = local write "DISP LAB01-1"(w694) -> ()
                      }
                      frame #4 {
                        n469 = local read "SIG LAB01-1"() -> (w698:T2)
                        n470 = local read "TEMP START LAB01-1"() -> (w700:cluster{"TL":dbl, "TN":dbl})
                        n471 = Unbundle(w698) -> ("Tmp Live"=w697:dbl, "Tmp Neut"=w696:dbl)  [unwired: 3 out]
                        n472 = Bundle(cluster=w700, "TL"=w697, "TN"=w696) -> (w699:cluster{"TL":dbl, "TN":dbl})
                        n473 = local write "TEMP START LAB01-1"(w699) -> ()
                      }
                    }
                  }
                }
              }
              event "RUN LAB01-2": Value Change {
                n474 = event-data() -> ("NewVal"=w701:bool)  [unwired: 1 in, 5 out]
                n475 = local write "run lab01-2"(w701) -> ()
                n476 = case shown="True" w701 {
                  tunnel: w707 -> [_ w740]
                  tunnel: w706 -> [_ w739]
                  tunnel: w704 -> [w709 w738]
                  tunnel: w705 -> [_ w737]
                  tunnel: w703 -> [_ w736]
                  tunnel: [w708 w735] -> w702
                  frame False {
                    # "stop test"
                    n477 = stacked-sequence {
                      tunnel: w709 -> [w718 _]
                      tunnel: [w710 _] -> w708
                      frame #0 {
                        n478 = local read "DISP LAB01-2"() -> (w717:T4)
                        n479 = Unbundle(w717) -> ("CYCLE"=w715:dbl, "MINS"=w716:dbl)  [unwired: 1 out]
                        n480 = case shown="\"CHART TEST\", Default" w718 {
                          tunnel: w716 -> [_ _ w725]
                          tunnel: w715 -> [w723 w724 _]
                          tunnel: [w723 w724 w725] -> w714
                          frame "CHART TEST", Default {
                          }
                          frame "CYCLE TEST" {
                          }
                          frame "T-RISE TEST" {
                          }
                        }
                        n481 = local read "TDMS LAB01-2"() -> (w722:refnum<k34>)
                        n482 = Build Array("STOPPED") -> (w719:string[])
                        n483 = Build Array(w714) -> (w713:dbl[])
                        n484 = TDMS Write(0:w722, 5:"TEST RESULT", 7:w719, 9:w713) -> (4:w711:refnum<k34>, 15:w712:errorcluster)  [unwired: 2 in, 2 out]
                        n485 = TDMS Close(8:w712, 11:w711) -> (0:w710:errorcluster)  [unwired: 1 out]
                      }
                      frame #1 {
                        n486 = local read "DISP LAB01-2"() -> (w729:T4)
                        n487 = stacked-sequence {
                          tunnel: "LAB01-2" -> [w731 w733]
                          frame #0 {
                            n488 = call "sub vi - defrag tdms v1.vi"("panel id"=w731) -> ("error out"=w730:errorcluster)  [unwired: 10 in]
                            n489 = local write "data file error"(w730) -> ()
                          }
                          frame #1 {
                            n490 = call "Save data file to network drive v1.vi"("panel id"=w733) -> ("network file save error"=w732:errorcluster)  [unwired: 9 in, 1 out]
                            n491 = local write "RESULT LAB01-2"(FALSE) -> ()
                            n492 = local write "data file error"(w732) -> ()
                          }
                        }
                        n493 = Bundle(cluster=w729, "STATUS"="STOP") -> (w727:T4)  [unwired: 2 in]
                        n494 = local write "DISP LAB01-2"(w727) -> ()
                      }
                    }
                  }
                  frame True {
                    # "start new test and create test file"
                    n495 = stacked-sequence {
                      seq-local: [w741 _ _ _ _] -> [_ w766 _ _ _]
                      tunnel: w740 -> [w746 _ _ _ _]
                      tunnel: w739 -> [w743 _ _ _ _]
                      tunnel: w738 -> [w756 _ _ _ _]
                      tunnel: w737 -> [w749 _ _ _ _]
                      tunnel: w736 -> [w744 _ _ _ _]
                      tunnel: [_ w760 _ _ _] -> w735
                      frame #0 {
                        w742 = "\\"
                        n496 = local read "SET LAB01-2"() -> (w751:T5)
                        n497 = case shown="\"CYCLE TEST\"" w756 {
                          tunnel: ["L01-2-CHART TEST-" "L01-2-CYCLE TEST-" "L01-2-T-RISE TEST-"] -> w752
                          frame "CHART TEST", Default {
                          }
                          frame "CYCLE TEST" {
                          }
                          frame "T-RISE TEST" {
                          }
                        }
                        n498 = Unbundle(w751) -> ("DESCRIPTION"=w750:string)  [unwired: 4 out]
                        n499 = Concatenate Strings(w746, "\\", w744, w742, w743, w742) -> (w753:string)
                        n500 = String To Path(string=w753) -> (path=w755:path)
                        n501 = Concatenate Strings(w753, w752, w750, "-", w749, ".tdms") -> (w741:string)
                        n502 = Create Folder(path (use dialog)=w755) -> (error out=w754:errorcluster)  [unwired: 2 in, 2 out]
                        n503 = global write "Global 1.vi" "LAB01-2 FILE"(w741) -> ()
                        n504 = call <vilib>:"Clear Errors.vi"("error in (no error)"=w754) -> ()  [unwired: 6 in, 1 out]
                      }
                      frame #1 {
                        n505 = String To Path(string=w766) -> (path=w761:path)
                        n506 = TDMS Open(5:FALSE, 6:FALSE, 10:T18."create or replace" ("operation (0:open)"), 11:w761) -> (0:w760:errorcluster, 3:→"TDMS LAB01-2":refnum<k34>)  [unwired: 3 in]
                      }
                      frame #2 {
                        n507 = local read "SET LAB01-2"() -> (w772:T5)
                        n508 = local read "TDMS LAB01-2"() -> (w783:refnum<k34>)
                        n509 = Build Array("Testers Name", "Description", "Set Test Cycles", "T-Rise minutes", "T-Rise Deg C") -> (w773:string[])
                        n510 = Unbundle(w772) -> ("NAME"=w771:string, "DESCRIPTION"=w770:string, "CYCLES"=w769:dbl, "T-RISE mins"=w768:dbl, "T-RISE deg C"=w767:dbl)
                        n511 = Number To Decimal String(number=w769) -> (decimal integer string=w782:string)  [unwired: 1 in]
                        n512 = Number To Decimal String(number=w768) -> (decimal integer string=w781:string)  [unwired: 1 in]
                        n513 = Number To Decimal String(number=w767) -> (decimal integer string=w780:string)  [unwired: 1 in]
                        n514 = Build Array(w771, w770, w782, w781, w780) -> (w779:string[])
                        n515 = TDMS Set Properties(5:w779, 7:w773, 11:w783) -> ()  [unwired: 3 in, 4 out]
                      }
                      frame #3 {
                        w785 = 0.0
                        n516 = local read "DISP LAB01-2"() -> (w787:T4)
                        n517 = Bundle(cluster=w787, "CYCLE"=w785, "MINS"=w785, "STATUS"="RUN") -> (w786:T4)
                        n518 = local write "DISP LAB01-2"(w786) -> ()
                      }
                      frame #4 {
                        n519 = local read "SIG LAB01-2"() -> (w790:T2)
                        n520 = local read "TEMP START LAB01-2"() -> (w792:cluster{"TL":dbl, "TN":dbl})
                        n521 = Unbundle(w790) -> ("Tmp Live"=w789:dbl, "Tmp Neut"=w788:dbl)  [unwired: 3 out]
                        n522 = Bundle(cluster=w792, "TL"=w789, "TN"=w788) -> (w791:cluster{"TL":dbl, "TN":dbl})
                        n523 = local write "TEMP START LAB01-2"(w791) -> ()
                      }
                    }
                  }
                }
              }
              event "RUN LAB02-1": Value Change {
                n524 = event-data() -> ("NewVal"=w793:bool)  [unwired: 1 in, 5 out]
                n525 = local write "run lab02-1"(w793) -> ()
                n526 = case shown="True" w793 {
                  tunnel: w799 -> [_ w832]
                  tunnel: w798 -> [_ w831]
                  tunnel: w796 -> [w801 w830]
                  tunnel: w797 -> [_ w829]
                  tunnel: w795 -> [_ w828]
                  tunnel: [w800 w827] -> w794
                  frame False {
                    # "stop test"
                    n527 = stacked-sequence {
                      tunnel: w801 -> [w810 _]
                      tunnel: [w802 _] -> w800
                      frame #0 {
                        n528 = local read "DISP LAB02-1"() -> (w809:T4)
                        n529 = Unbundle(w809) -> ("CYCLE"=w807:dbl, "MINS"=w808:dbl)  [unwired: 1 out]
                        n530 = case shown="\"CYCLE TEST\"" w810 {
                          tunnel: w808 -> [_ _ w817]
                          tunnel: w807 -> [w815 w816 _]
                          tunnel: [w815 w816 w817] -> w806
                          frame "CHART TEST", Default {
                          }
                          frame "CYCLE TEST" {
                          }
                          frame "T-RISE TEST" {
                          }
                        }
                        n531 = local read "TDMS LAB02-1"() -> (w814:refnum<k34>)
                        n532 = Build Array("STOPPED") -> (w811:string[])
                        n533 = Build Array(w806) -> (w805:dbl[])
                        n534 = TDMS Write(0:w814, 5:"TEST RESULT", 7:w811, 9:w805) -> (4:w803:refnum<k34>, 15:w804:errorcluster)  [unwired: 2 in, 2 out]
                        n535 = TDMS Close(8:w804, 11:w803) -> (0:w802:errorcluster)  [unwired: 1 out]
                      }
                      frame #1 {
                        n536 = local read "DISP LAB02-1"() -> (w821:T4)
                        n537 = stacked-sequence {
                          tunnel: "LAB02-1" -> [w823 w825]
                          frame #0 {
                            n538 = call "sub vi - defrag tdms v1.vi"("panel id"=w823) -> ("error out"=w822:errorcluster)  [unwired: 10 in]
                            n539 = local write "data file error"(w822) -> ()
                          }
                          frame #1 {
                            n540 = local write "RESULT LAB02-1"(FALSE) -> ()
                            n541 = call "Save data file to network drive v1.vi"("panel id"=w825) -> ("network file save error"=w824:errorcluster)  [unwired: 9 in, 1 out]
                            n542 = local write "data file error"(w824) -> ()
                          }
                        }
                        n543 = Bundle(cluster=w821, "STATUS"="STOP") -> (w819:T4)  [unwired: 2 in]
                        n544 = local write "DISP LAB02-1"(w819) -> ()
                      }
                    }
                  }
                  frame True {
                    # "start new test and create test file"
                    n545 = stacked-sequence {
                      seq-local: [w833 _ _ _ _] -> [_ w858 _ _ _]
                      tunnel: w832 -> [w838 _ _ _ _]
                      tunnel: w831 -> [w835 _ _ _ _]
                      tunnel: w830 -> [w848 _ _ _ _]
                      tunnel: w829 -> [w841 _ _ _ _]
                      tunnel: w828 -> [w836 _ _ _ _]
                      tunnel: [_ w852 _ _ _] -> w827
                      frame #0 {
                        w834 = "\\"
                        n546 = local read "SET LAB02-1"() -> (w843:T5)
                        n547 = case shown="\"CYCLE TEST\"" w848 {
                          tunnel: ["L02-1-CHART TEST-" "L02-1-CYCLE TEST-" "L02-1-T-RISE TEST-"] -> w844
                          frame "CHART TEST", Default {
                          }
                          frame "CYCLE TEST" {
                          }
                          frame "T-RISE TEST" {
                          }
                        }
                        n548 = Unbundle(w843) -> ("DESCRIPTION"=w842:string)  [unwired: 4 out]
                        n549 = Concatenate Strings(w838, "\\", w836, w834, w835, w834) -> (w845:string)
                        n550 = String To Path(string=w845) -> (path=w847:path)
                        n551 = Concatenate Strings(w845, w844, w842, "-", w841, ".tdms") -> (w833:string)
                        n552 = Create Folder(path (use dialog)=w847) -> (error out=w846:errorcluster)  [unwired: 2 in, 2 out]
                        n553 = global write "Global 1.vi" "LAB02-1 FILE"(w833) -> ()
                        n554 = call <vilib>:"Clear Errors.vi"("error in (no error)"=w846) -> ()  [unwired: 6 in, 1 out]
                      }
                      frame #1 {
                        n555 = String To Path(string=w858) -> (path=w853:path)
                        n556 = TDMS Open(5:FALSE, 6:FALSE, 10:T18."create or replace" ("operation (0:open)"), 11:w853) -> (0:w852:errorcluster, 3:→"TDMS LAB02-1":refnum<k34>)  [unwired: 3 in]
                      }
                      frame #2 {
                        n557 = local read "SET LAB02-1"() -> (w864:T5)
                        n558 = local read "TDMS LAB02-1"() -> (w875:refnum<k34>)
                        n559 = Build Array("Testers Name", "Description", "Set Test Cycles", "T-Rise minutes", "T-Rise Deg C") -> (w865:string[])
                        n560 = Unbundle(w864) -> ("NAME"=w863:string, "DESCRIPTION"=w862:string, "CYCLES"=w861:dbl, "T-RISE mins"=w860:dbl, "T-RISE deg C"=w859:dbl)
                        n561 = Number To Decimal String(number=w861) -> (decimal integer string=w874:string)  [unwired: 1 in]
                        n562 = Number To Decimal String(number=w860) -> (decimal integer string=w873:string)  [unwired: 1 in]
                        n563 = Number To Decimal String(number=w859) -> (decimal integer string=w872:string)  [unwired: 1 in]
                        n564 = Build Array(w863, w862, w874, w873, w872) -> (w871:string[])
                        n565 = TDMS Set Properties(5:w871, 7:w865, 11:w875) -> ()  [unwired: 3 in, 4 out]
                      }
                      frame #3 {
                        w877 = 0.0
                        n566 = local read "DISP LAB02-1"() -> (w879:T4)
                        n567 = Bundle(cluster=w879, "CYCLE"=w877, "MINS"=w877, "STATUS"="RUN") -> (w878:T4)
                        n568 = local write "DISP LAB02-1"(w878) -> ()
                      }
                      frame #4 {
                        n569 = local read "SIG LAB02-1"() -> (w882:T2)
                        n570 = local read "TEMP START LAB02-1"() -> (w884:cluster{"TL":dbl, "TN":dbl})
                        n571 = Unbundle(w882) -> ("Tmp Live"=w881:dbl, "Tmp Neut"=w880:dbl)  [unwired: 3 out]
                        n572 = Bundle(cluster=w884, "TL"=w881, "TN"=w880) -> (w883:cluster{"TL":dbl, "TN":dbl})
                        n573 = local write "TEMP START LAB02-1"(w883) -> ()
                      }
                    }
                  }
                }
              }
              event "RUN LAB02-2": Value Change {
                n574 = event-data() -> ("NewVal"=w885:bool)  [unwired: 1 in, 5 out]
                n575 = local write "run lab02-2"(w885) -> ()
                n576 = case shown="True" w885 {
                  tunnel: w891 -> [_ w924]
                  tunnel: w890 -> [_ w923]
                  tunnel: w888 -> [w893 w922]
                  tunnel: w889 -> [_ w921]
                  tunnel: w887 -> [_ w920]
                  tunnel: [w892 w919] -> w886
                  frame False {
                    # "stop test"
                    n577 = stacked-sequence {
                      tunnel: w893 -> [w902 _]
                      tunnel: [w894 _] -> w892
                      frame #0 {
                        n578 = local read "DISP LAB02-2"() -> (w901:T4)
                        n579 = Unbundle(w901) -> ("CYCLE"=w899:dbl, "MINS"=w900:dbl)  [unwired: 1 out]
